vi "Write Line Data.vi"(6 "end point":i32, 7 "start point":i32, 8 "error in (no error)":errorcluster, 9 "end value":i32, 10 "start value":i32, 11 "VISA resource name":refnum<visa-resource-name>) -> (0 "error out":errorcluster, 3 "VISA resource name out":refnum<visa-resource-name>)   [LabVIEW 2009, in "Tektronix AFG 3000 Series.lvlib"]
doc: "Writes line data to the edit memory of a Tektronix AFG 3000 series function generator. You specify the starting point and value, and the ending point and value, and the AFG linearly interpolates in between."
uses:
  Tektronix AFG 3000 Series.lvlib
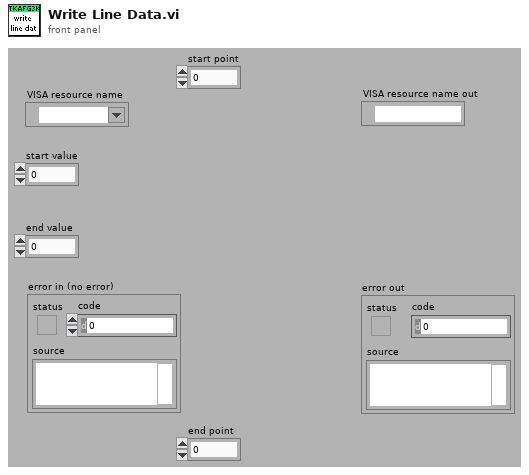
[diagram p1: front panel]
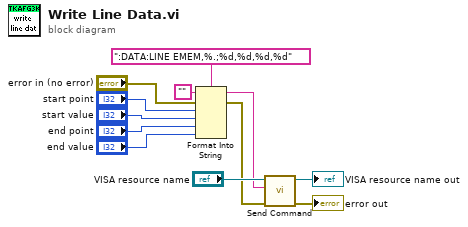
[diagram p0: block diagram]
diagram:
  n1 = Format Into String(format string=":DATA:LINE EMEM,%.;%d,%d,%d,%d", initial string="", error in="error in (no error)", "start point", "start value", "end point", "end value") -> (resulting string=w10:string, error out=w8:errorcluster)
  n2 = call "Send Command.vi"("error in (no error)"=w8, "write buffer"=w10, "VISA resource name"="VISA resource name") -> ("error out"=→"error out":errorcluster, "VISA resource name out"=→"VISA resource name out":refnum<visa-resource-name>)  [unwired: 7 out]
